vi "demo_getdi.vi"() -> ()   [LabVIEW 2017]
panel:
  out "数字":i32 format="%x"
  in  "name":string="mrx-t4"
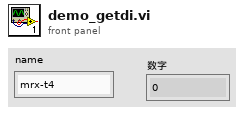
[diagram p1: front panel]
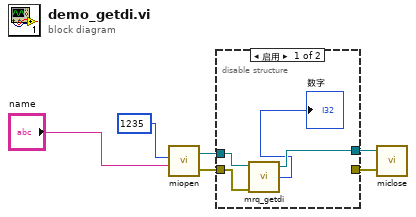
[diagram p0: block diagram]
diagram:
  n1 = call "miopen.vi"("name"="name", "port"=u16 1235) -> ("错误输出"=w3:errorcluster, "VISA资源名称输出"=w6:refnum<visa-resource-name>)  [unwired: 2 in]
  n2 = disable-structure shown="启用" {
    disable-tunnel: w6 -> [w10 w12]
    disable-tunnel: [w8 w12] -> w5
    disable-tunnel: [_ w11] -> w4
    disable-tunnel: w3 -> [w9 w11]
    frame Enabled {
      n3 = call "mrq_getdi.vi"("错误输入（无错误）"=w9, "VISA资源名称"=w10) -> ("数字"=→"数字":i32, "VISA资源名称输出"=w8:refnum<visa-resource-name>)  [unwired: 2 in, 1 out]
    }
    frame Disabled {
    }
  }
  n4 = call "miclose.vi"("错误输入（无错误）"=w4, "VISA资源名称"=w5) -> ()  [unwired: 1 out]
